vi "LiftZero.vi"(10 "LiftZeroOverride":bool) -> ()   [LabVIEW 2014, in "LiftLib.lvlib"]
uses:
  LiftLib.lvlib
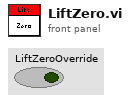
[diagram p1: front panel]
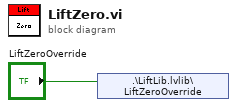
[diagram p0: block diagram]
diagram:
  n1 = shared-variable ".\\LiftLib.lvlib\\LiftZeroOverride"("LiftZeroOverride") -> ()  [unwired: 1 in, 1 out]
